vi "Recieve Calibration.vi"(8 "error in (no error)":errorcluster, 11 "RP Communicator in":refnum<class "RP Communicator.lvclass">) -> (0 "error out":errorcluster, 2 "Calibration":T1 {"magic" format="%x"}, 3 "RP Communicator out":refnum<class "RP Communicator.lvclass">)   [LabVIEW 2024, in "RP Communicator.lvclass"]
uses:
  RP Communicator.lvclass
  RP EEPROM Calibration.ctl
  RP Command.ctl
  RP Communicator.lvclass/RP Communicator.ctl
  Write RP EEPROM Calibration.vi
  Read RP EEPROM Calibration.vi
  Read Timeout.vi
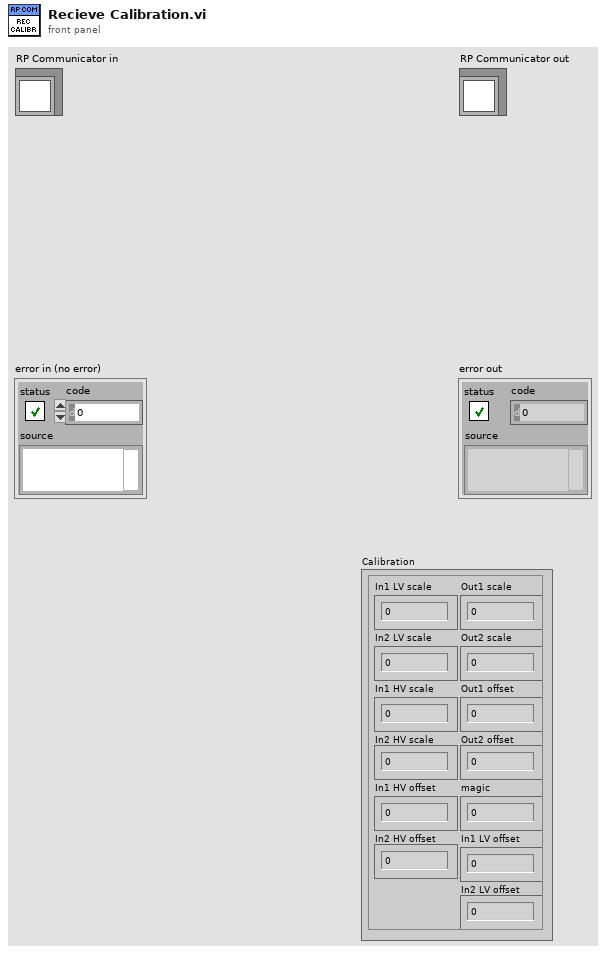
[diagram p1: front panel]
types:
  T1 = typedef "RP EEPROM Calibration.ctl" = cluster{"In1 LV scale":u32, "In2 LV scale":u32, "In1 HV scale":u32, "In2 HV scale":u32, "In1 HV offset":i32, "In2 HV offset":i32, "Out1 scale":u32, "Out2 scale":u32, "Out1 offset":i32, "Out2 offset":i32, "magic":u32, "In1 LV offset":i32, "In2 LV offset":i32}
  T2 = typedef "RP Command.ctl" = enum16{"Reset", "Read IDN", "Stop server", "Get status", "Get temperature", "Connect client", "Arm", "Software trigger", "Get whole buffer", "Get chunk", "System call", "Get config", "Set config", "Recieve data", "Recieve Calibartion", "Transmit data"}
  T3 = enum16{"big-endian, network order", "native, host order", "little-endian"}
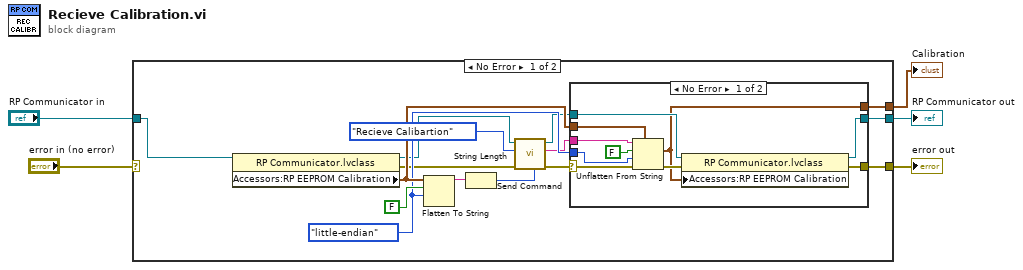
[diagram p0: block diagram]
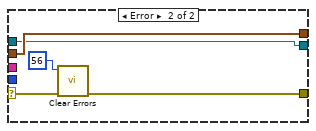
[diagram p2: hidden frame]
diagram:
  n1 = case shown="No Error" "error in (no error)" {
    selector: "error in (no error)" -> [_ w37]
    tunnel: [w19 w37] -> w4
    tunnel: [w18 w36] -> w2
    tunnel: "RP Communicator in" -> [w10 w36]
    tunnel: [w17 _] -> w1
    frame No Error {
      w13 = T3."little-endian" ("byte order (0:big-endian, network order)")
      n2 = property class="RP Communicator.lvclass"(reference=w10) -> (reference out=w11:refnum<class "RP Communicator.lvclass">, error out=w8:errorcluster, "Accessors:RP EEPROM Calibration"=w14:T1)  [unwired: 1 in]
      n3 = Flatten To String(anything=w14, prepend array or string size? (T)=FALSE, byte order (0:big-endian, network order)=w13) -> (data string=w15:string)  [unwired: 1 in, 2 out]
      n4 = String Length(string=w15) -> (length=w6:i32)
      n5 = call-dynamic "Send Command.vi"("bytes to read"=w6, "error in (no error)"=w8, "Command number"=RP_Command."Recieve Calibartion", "RP Communicator in"=w11) -> ("error out"=w9:errorcluster, "data out"=w7:string, "RP Communicator out"=w12:refnum<class "RP Communicator.lvclass">)  [unwired: 5 in]
      n6 = case shown="No Error" w9 {
        selector: w9 -> [w21 w35]
        tunnel: w12 -> [w30 w31]
        tunnel: w7 -> [w28 _]
        tunnel: [w26 w33] -> w19
        tunnel: [w25 w31] -> w18
        tunnel: [w24 w34] -> w17
        tunnel: w14 -> [w23 w34]
        tunnel: w13 -> [w22 _]
        frame No Error {
          n7 = Unflatten From String(type=w23, binary string=w28, data includes array or string size? (T)=FALSE, byte order (0:big-endian, network order)=w22, error in (no error)=w21) -> (value=w24:T1, error out=w27:errorcluster)  [unwired: 1 out]
          n8 = property class="RP Communicator.lvclass"(reference=w30, error in=w27, "Accessors:RP EEPROM Calibration"=w24) -> (reference out=w25:refnum<class "RP Communicator.lvclass">, error out=w26:errorcluster)
        }
        frame Error {
          n9 = call <vilib>:"Clear Errors.vi"("error in (no error)"=w35, "specific error code to clear (0: all)"=56) -> ("error out"=w33:errorcluster)  [unwired: 4 in, 1 out]
        }
      }
    }
    frame Error {
    }
  }
  "error out" <- w4
  "RP Communicator out" <- w2
  "Calibration" <- w1
